vi "Project Initializer - Update Project Name Constant VI.vi"(8 "error in (no error)":errorcluster, 10 "New Project Name":string, 11 "New Project _Source Directory":path) -> (0 "error out":errorcluster)   [LabVIEW 2022 SP3]
uses:
  <vilib>/Utility/traverseref.llb/TRef TravTarget.ctl
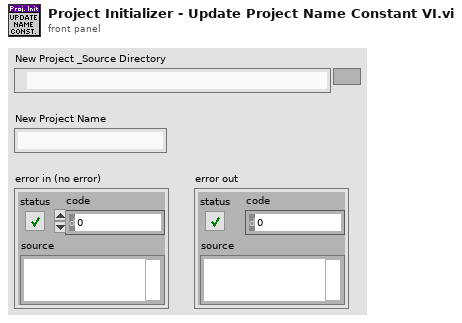
[diagram p1: front panel]
types:
  T1 = typedef "TRef TravTarget.ctl" = enum16{"FP", "BD", "Other"}
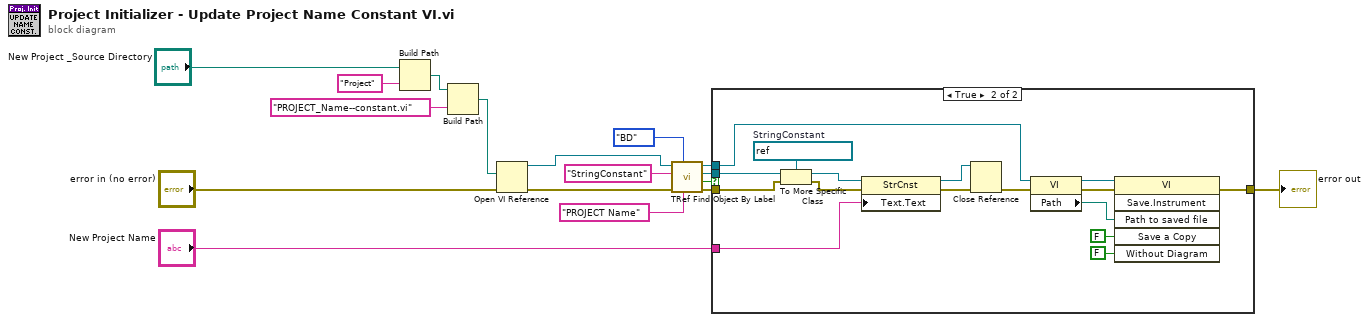
[diagram p0: block diagram]
diagram:
  n1 = Build Path(base path="New Project _Source Directory", name or relative path="Project") -> (appended path=w5:path)
  n2 = Build Path(base path=w5, name or relative path="PROJECT_Name--constant.vi") -> (appended path=w4:path)
  n3 = Open VI Reference(vi path=w4, error in (no error)="error in (no error)") -> (vi reference=w9:refnum<vi>, error out=w10:errorcluster)  [unwired: 4 in]
  n4 = call <vilib>:"TRef Find Object By Label.vi"("Label"="PROJECT Name", "Traverse Target"=TRef_TravTarget."BD", "error in (no error)"=w10, "Class Name"="StringConstant", "VI Ref"=w9) -> ("error out"=w14:errorcluster, "Found?"=w17:bool, "Found Obj Ref"=w13:refnum<vi>, "dup VI Ref"=w15:refnum<vi>)  [unwired: 3 in]
  n5 = case shown="True" w17 {
    tunnel: w13 -> [_ w33]
    tunnel: w14 -> [w18 w28]
    tunnel: w15 -> [_ w27]
    tunnel: [w18 w25] -> w1
    tunnel: "New Project Name" -> [_ w19]
    frame False {
    }
    frame True {
      w34 = refnum<vi> refnum  # StringConstant
      n6 = To More Specific Class(target class=w34, reference=w33, error in=w28) -> (specific class reference=w32:refnum<vi>, error out=w31:errorcluster)
      n7 = property class="StrCnst"(reference=w32, error in=w31, "Text.Text"=w19) -> (reference out=w22:refnum<vi>, error out=w24:errorcluster)
      n8 = Close Reference(reference=w22, error in (no error)=w24) -> (error out=w21:errorcluster)
      n9 = property class="VI"(reference=w27, error in=w21) -> (reference out=w26:refnum<vi>, error out=w20:errorcluster, "Path"=w23:path)
      n10 = invoke class="VI" method="Save.Instrument"(reference=w26, error in=w20, "Path to saved file"=w23, "Save a Copy"=FALSE, "Without Diagram"=FALSE) -> (error out=w25:errorcluster)  [unwired: 1 in, 5 out]
    }
  }
  "error out" <- w1
